vi "Calc_Moments.vi"(5 "Number of Cores":i32=4, 6 "Pre-Calc-Array":cluster{"X2":sgl[], "Y2":sgl[], "XY":sgl[][]}={"X2"=[1.0, 4.0, 9.0, 16.0, 25.0, 36.0, 49.0, 64.0, 81.0, 100.0, 121.0, 144.0, 169.0, 196.0, 225.0, 256.0, 289.0, 324.0, 361.0, 400.0, 441.0, 484.0, 529.0, 576.0, 625.0, 676.0, 729.0, 784.0, 841.0, 900.0, 961.0, 1024.0, 1089.0, 1156.0, 1225.0, 1296.0, 1369.0, 1444.0, 1521.0, 1600.0, 1681.0, 1764.0, 1849.0, 1936.0, 2025.0, 2116.0, 2209.0, 2304.0, 2401.0, 2500.0, 2601.0, 2704.0, 2809.0, 2916.0, 3025.0, 3136.0, 3249.0, 3364.0, 3481.0, 3600.0, 3721.0, 3844.0, 3969.0, 4096.0, 4225.0, 4356.0, 4489.0, 4624.0, 4761.0, 4900.0, 5041.0, 5184.0, 5329.0, 5476.0, 5625.0, 5776.0, 5929.0, 6084.0, 6241.0, 6400.0, 6561.0, 6724.0, 6889.0, 7056.0, 7225.0, 7396.0, 7569.0, 7744.0, 7921.0, 8100.0, 8281.0, 8464.0, 8649.0, 8836.0, 9025.0, 9216.0, 9409.0, 9604.0, 9801.0, 10000.0], "Y2"=[1.0, 4.0, 9.0, 16.0, 25.0, 36.0, 49.0, 64.0, 81.0, 100.0, 121.0, 144.0, 169.0, 196.0, 225.0, 256.0, 289.0, 324.0, 361.0, 400.0, 441.0, 484.0, 529.0, 576.0, 625.0, 676.0, 729.0, 784.0, 841.0, 900.0, 961.0, 1024.0, 1089.0, 1156.0, 1225.0, 1296.0, 1369.0, 1444.0, 1521.0, 1600.0, 1681.0, 1764.0, 1849.0, 1936.0, 2025.0, 2116.0, 2209.0, 2304.0, 2401.0, 2500.0, 2601.0, 2704.0, 2809.0, 2916.0, 3025.0, 3136.0, 3249.0, 3364.0, 3481.0, 3600.0, 3721.0, 3844.0, 3969.0, 4096.0, 4225.0, 4356.0, 4489.0, 4624.0, 4761.0, 4900.0, 5041.0, 5184.0, 5329.0, 5476.0, 5625.0, 5776.0, 5929.0, 6084.0, 6241.0, 6400.0, 6561.0, 6724.0, 6889.0, 7056.0, 7225.0, 7396.0, 7569.0, 7744.0, 7921.0, 8100.0, 8281.0, 8464.0, 8649.0, 8836.0, 9025.0, 9216.0, 9409.0, 9604.0, 9801.0, 10000.0], "XY"=array100x100[10000 elements]}, 11 "Image Pixels (single)":sgl[][](array[numeric])) -> (0 "Minor Axis":dbl=0.2950867911863983, 1 "Major Axis":dbl=0.2950867911863983, 2 "Major Angle":dbl=0.2950867911863983, 3 "Centroid":cluster{"X":dbl, "Y":dbl}={"X"=71.90286041423869, "Y"=56.08303175284713})   [LabVIEW 2014]
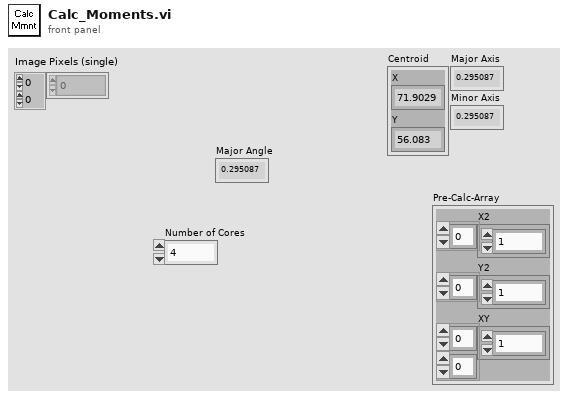
[diagram p1: front panel]
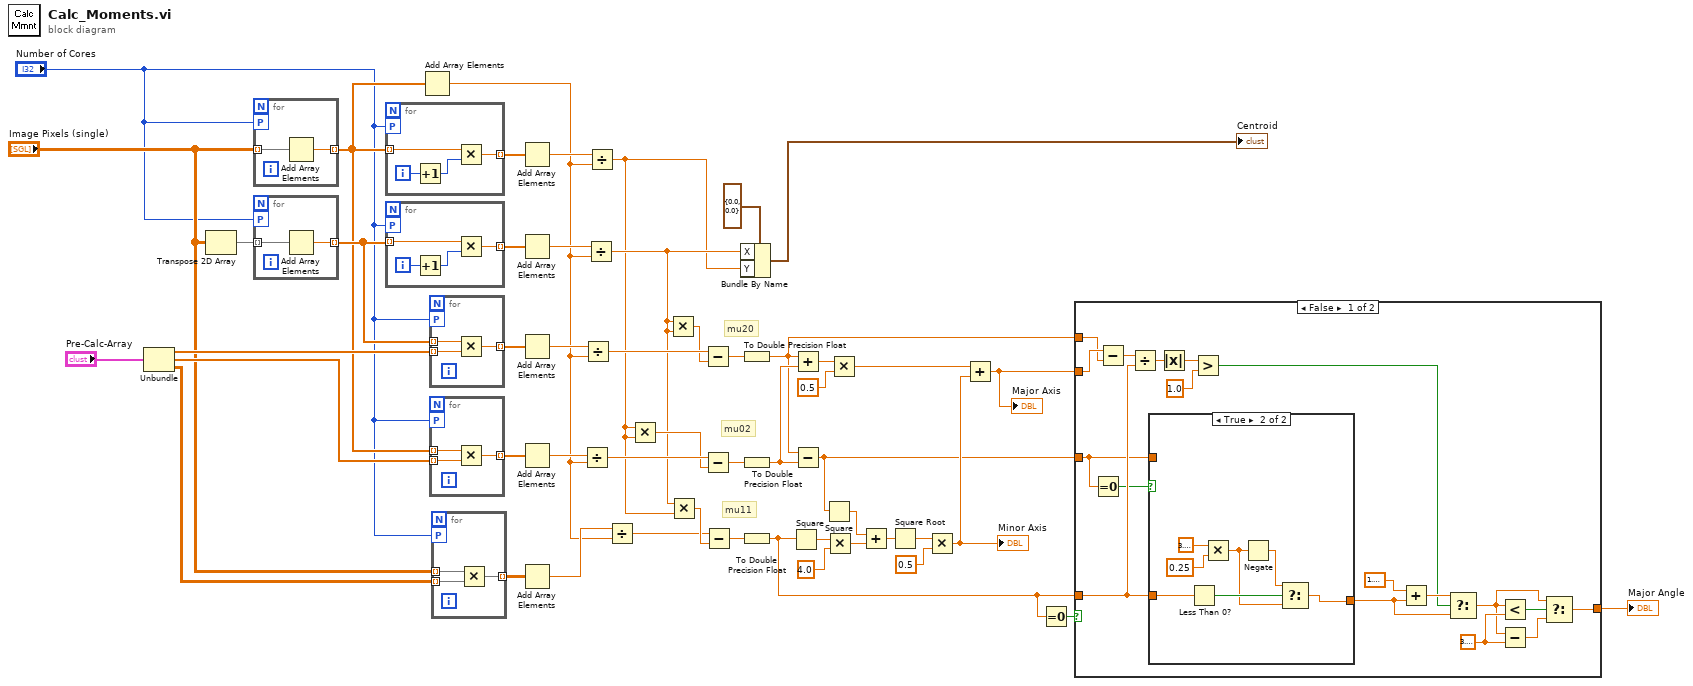
[diagram p0: block diagram]
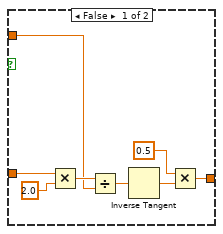
[diagram p2: hidden frame]
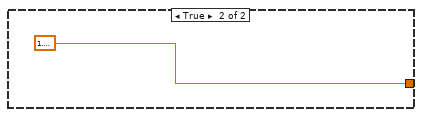
[diagram p3: hidden frame]
diagram:
  # "mu11"
  # "mu02"
  # "mu20"
  n1 = Unbundle("Pre-Calc-Array") -> ("X2"=w36:sgl[], "Y2"=w44:sgl[], "XY"=w43:sgl[][])
  n2 = Transpose 2D Array(2D array="Image Pixels (single)") -> (transposed array=w49:sgl[][])
  n3 = for {
    tunnel: "Image Pixels (single)" -> [w53] mode=indexing
    tunnel: [w52] -> w35 mode=indexing
    workers-P: "Number of Cores" -> [_]
    n4 = Add Array Elements(numeric array=w53) -> (sum=w52:sgl)
  }
  n5 = for {
    tunnel: w49 -> [w55] mode=indexing
    tunnel: [w54] -> w37 mode=indexing
    workers-P: "Number of Cores" -> [_]
    n6 = Add Array Elements(numeric array=w55) -> (sum=w54:sgl)
  }
  n7 = for {
    tunnel: w35 -> [w57] mode=indexing
    tunnel: [w56] -> w48 mode=indexing
    workers-P: "Number of Cores" -> [_]
    i -> [w59]
    n8 = Increment(x=w59) -> (x+1=w58:i32)
    n9 = Multiply(x=w57, y=w58) -> (x*y=w56:sgl)
  }
  n10 = for {
    tunnel: w37 -> [w61] mode=indexing
    tunnel: [w60] -> w47 mode=indexing
    workers-P: "Number of Cores" -> [_]
    i -> [w63]
    n11 = Increment(x=w63) -> (x+1=w62:i32)
    n12 = Multiply(x=w61, y=w62) -> (x*y=w60:sgl)
  }
  n13 = Add Array Elements(numeric array=w35) -> (sum=w29:sgl)
  n14 = for {
    tunnel: [w66] -> w46 mode=indexing
    tunnel: w36 -> [w65] mode=indexing
    tunnel: w37 -> [w64] mode=indexing
    workers-P: "Number of Cores" -> [_]
    n15 = Multiply(x=w64, y=w65) -> (x*y=w66:sgl)
  }
  n16 = for {
    tunnel: [w69] -> w45 mode=indexing
    tunnel: w44 -> [w68] mode=indexing
    tunnel: w35 -> [w67] mode=indexing
    workers-P: "Number of Cores" -> [_]
    n17 = Multiply(x=w67, y=w68) -> (x*y=w69:sgl)
  }
  n18 = for {
    tunnel: w43 -> [w72] mode=indexing
    tunnel: [w71] -> w42 mode=indexing
    tunnel: "Image Pixels (single)" -> [w70] mode=indexing
    workers-P: "Number of Cores" -> [_]
    n19 = Multiply(x=w70, y=w72) -> (x*y=w71:sgl[])
  }
  n20 = Add Array Elements(numeric array=w48) -> (sum=w41:sgl)
  n21 = Add Array Elements(numeric array=w47) -> (sum=w40:sgl)
  n22 = Add Array Elements(numeric array=w46) -> (sum=w39:sgl)
  n23 = Add Array Elements(numeric array=w45) -> (sum=w31:sgl)
  n24 = Add Array Elements(numeric array=w42) -> (sum=w30:sgl)
  n25 = Divide(x=w31, y=w29) -> (x/y=w33:sgl)
  n26 = Divide(x=w39, y=w29) -> (x/y=w38:sgl)
  n27 = Divide(x=w40, y=w29) -> (x/y=w25:sgl)
  n28 = Divide(x=w41, y=w29) -> (x/y=w24:sgl)
  n29 = Divide(x=w30, y=w29) -> (x/y=w27:sgl)
  n30 = Multiply(x=w24, y=w24) -> (x*y=w32:sgl)
  n31 = Multiply(x=w25, y=w25) -> (x*y=w34:sgl)
  n32 = Multiply(x=w25, y=w24) -> (x*y=w28:sgl)
  n33 = Subtract(x=w38, y=w34) -> (x-y=w21:sgl)
  n34 = Subtract(x=w33, y=w32) -> (x-y=w20:sgl)
  n35 = Subtract(x=w27, y=w28) -> (x-y=w19:sgl)
  n36 = Bundle By Name(cluster=cluster{"X":dbl, "Y":dbl} {"X"=0.0, "Y"=0.0} ("Start Point"), "X"=w25, "Y"=w24) -> (→"Centroid":cluster{"X":dbl, "Y":dbl})
  n37 = To Double Precision Float(number=w21) -> (double precision float=w5:dbl)
  n38 = To Double Precision Float(number=w20) -> (double precision float=w18:dbl)
  n39 = To Double Precision Float(number=w19) -> (double precision float=w1:dbl)
  n40 = Square(x=w1) -> (x^2=w15:dbl)
  n41 = Add(x=w5, y=w18) -> (x+y=w17:dbl)
  n42 = Subtract(x=w5, y=w18) -> (x-y=w3:dbl)
  n43 = Square(x=w3) -> (x^2=w13:dbl)
  n44 = Multiply(x=w15, y=4.0) -> (x*y=w12:dbl)
  n45 = Multiply(x=w17, y=0.5) -> (x*y=w8:dbl)
  n46 = Add(x=w13, y=w12) -> (x+y=w11:dbl)
  n47 = Square Root(x=w11) -> (sqrt(x)=w9:dbl)
  n48 = Multiply(x=w9, y=0.5) -> (x*y=w7:dbl)
  "Minor Axis" <- w7
  n49 = Add(x=w8, y=w7) -> (x+y=w6:dbl)
  "Major Axis" <- w6
  n50 = Equal To 0?(x=w1) -> (x = 0?=w2:bool)
  n51 = case shown="False" w2 {
    tunnel: w6 -> [w90 _]
    tunnel: w5 -> [w89 _]
    tunnel: [w73 1.5707963267948966] -> w4
    tunnel: w1 -> [w86 _]
    tunnel: w3 -> [w84 _]
    frame False {
      w78 = 3.141592653589793
      n52 = Equal To 0?(x=w84) -> (x = 0?=w85:bool)
      n53 = Subtract(x=w90, y=w89) -> (x-y=w88:dbl)
      n54 = Divide(x=w88, y=w86) -> (x/y=w87:dbl)
      n55 = case shown="True" w85 {
        tunnel: w86 -> [w97 w105]
        tunnel: [w91 w99] -> w77
        tunnel: w84 -> [w95 _]
        frame False {
          n56 = Multiply(x=w97, y=2.0) -> (x*y=w96:dbl)
          n57 = Divide(x=w96, y=w95) -> (x/y=w94:dbl)
          n58 = Inverse Tangent(1:w94) -> (0:w93:dbl)
          n59 = Multiply(x=0.5 ("y"), y=w93) -> (x*y=w91:dbl)
        }
        frame True {
          n60 = Less Than 0?(x=w105) -> (x < 0?=w102:bool)
          n61 = Multiply(x=3.141592653589793, y=0.25) -> (x*y=w100:dbl)
          n62 = Negate(x=w100) -> (-x=w101:dbl)
          n63 = Select(t=w101, s=w102, f=w100) -> (s? t:f=w99:dbl)
        }
      }
      n64 = Absolute Value(x=w87) -> (abs(x)=w82:dbl)
      n65 = Greater?(x=w82, y=1.0) -> (0:w79:bool)
      n66 = Add(x=1.5707963267948966, y=w77) -> (x+y=w80:dbl)
      n67 = Select(t=w80, s=w79, f=w77) -> (s? t:f=w75:dbl)
      n68 = Less?(x=w75, y=w78) -> (x < y?=w76:bool)
      n69 = Subtract(x=w75, y=w78) -> (x-y=w74:dbl)
      n70 = Select(t=w75, s=w76, f=w74) -> (s? t:f=w73:dbl)
    }
    frame True {
    }
  }
  "Major Angle" <- w4
